vi "Joystick.vi"(11 "Enum":enum16{"Start", "Run", "End"}(ring)) -> (1 "Buttons":bool[](array[boolean]), 2 "Axes":dbl[](array[numeric]))   [LabVIEW 2014]
uses:
  <vilib>/Rock Robotics/WPI/Joystick/WPI_JoystickDeviceEnum.ctl
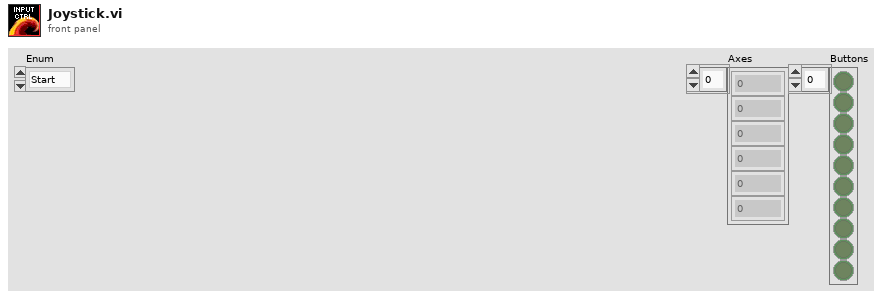
[diagram p1: front panel]
types:
  T1 = typedef "WPI_JoystickDeviceEnum.ctl" = enum16{"USB 0", "USB 1", "USB 2", "USB 3", "USB 4", "USB 5"}
  T2 = typedef "WPI_JoystickDevRef.ctl" = cluster{"Device":T1}
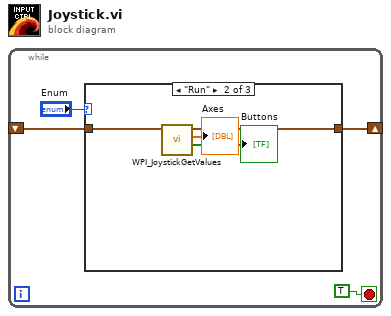
[diagram p0: block diagram]
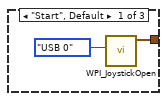
[diagram p2: hidden frame]
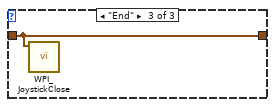
[diagram p3: hidden frame]
diagram:
  n1 = while {
    shift-right: [w3] -> _
    shift-left: _ -> [w1]
    stop <- TRUE stop-if-true
    n2 = case shown="\"Run\"" "Enum" {
      tunnel: [w6 w9 w11] -> w3
      tunnel: w1 -> [_ w10 w11]
      frame "Start", Default {
        n3 = call <vilib>:"WPI_JoystickOpen.vi"("JoystickDevice"=WPI_JoystickDeviceEnum."USB 0") -> ("JoystickDevRef"=w6:T2)  [unwired: 10 in]
      }
      frame "Run" {
        n4 = call <vilib>:"WPI_JoystickGetValues.vi"("JoystickDevRef"=w10) -> ("Buttons"=→"Buttons":bool[], "Axes"=→"Axes":dbl[], "JoystickDevRef"=w9:T2)  [unwired: 6 in, 2 out]
      }
      frame "End" {
        n5 = call <vilib>:"WPI_JoystickClose.vi"("JoystickDevRef"=w11) -> ()  [unwired: 11 in]
      }
    }
  }
